vi "do_GB_test.vi"(8 "error in (no error)":errorcluster, 11 "VISA resource name":refnum<visa-resource-name>="COM6") -> (0 "error out":errorcluster, 1 "Results GB":string, 2 "Status GB":string, 3 "VISA resource out":refnum<visa-resource-name>)   [LabVIEW 2015]
doc: "Mini test app for SERIAL RS232 or GPIB communication ports"
uses:
  Type Definitions/Highway_GB_Data.ctl
panel:
  # "Do GB test"
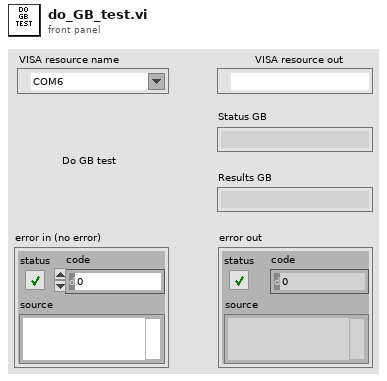
[diagram p1: front panel]
types:
  T1 = typedef "Highway_GB_Data.ctl" = cluster{"Status GB":string, "Results GB":string}
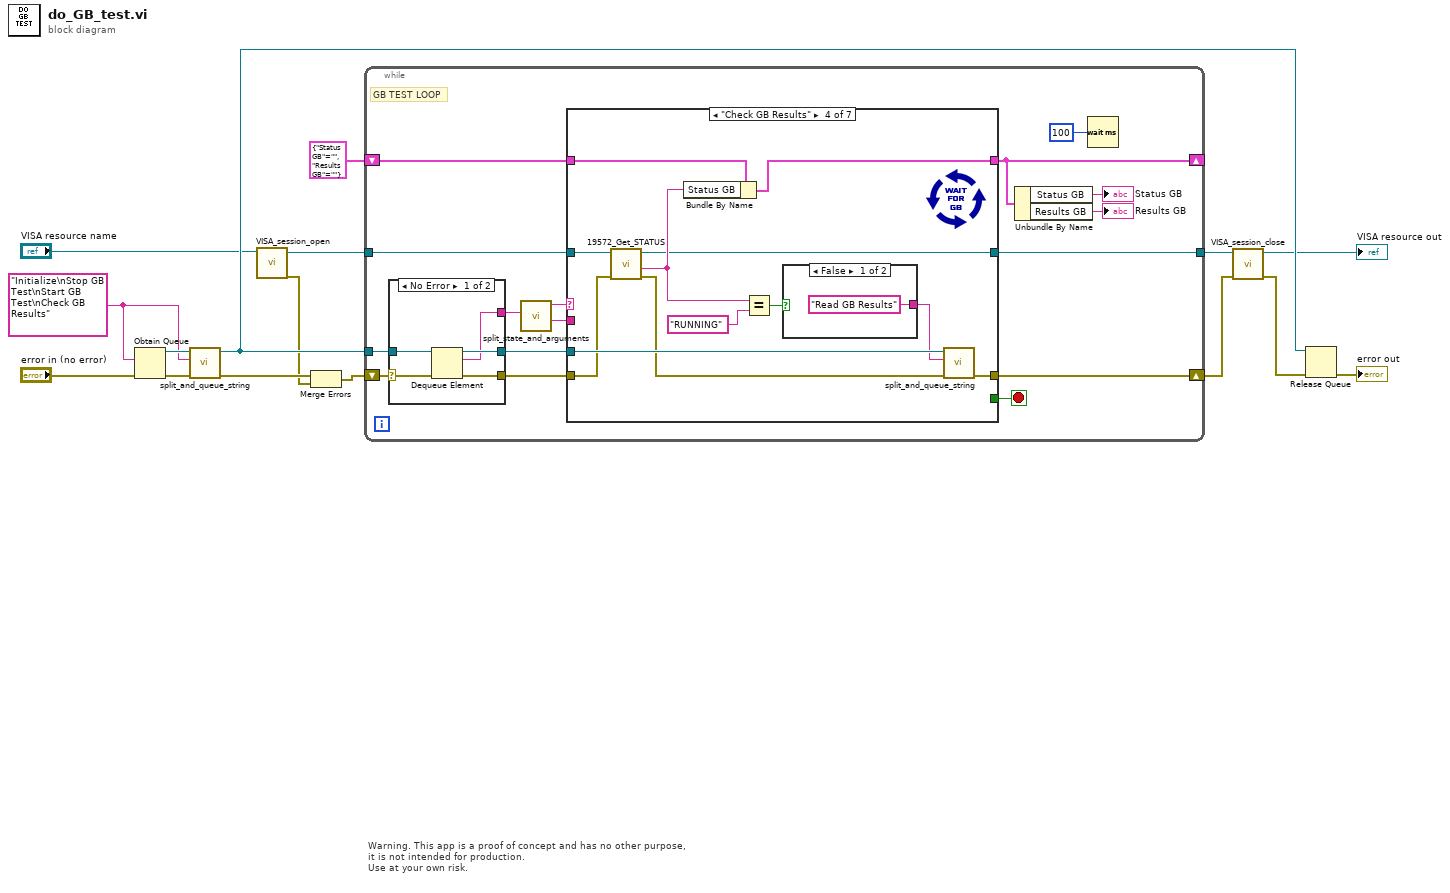
[diagram p0: block diagram]
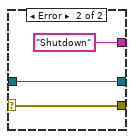
[diagram p2: hidden frame]
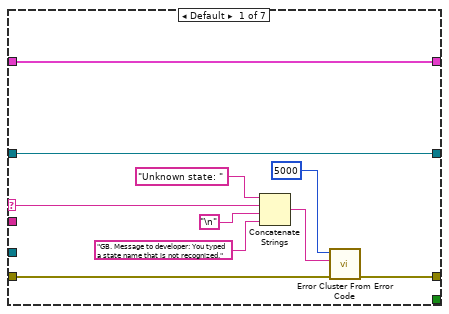
[diagram p3: hidden frame]
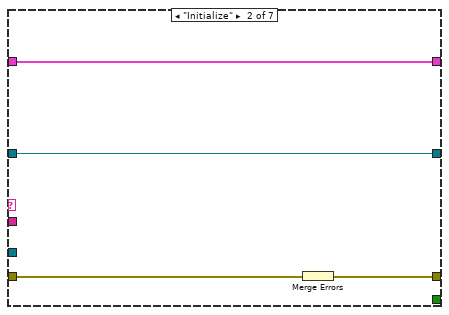
[diagram p4: hidden frame]
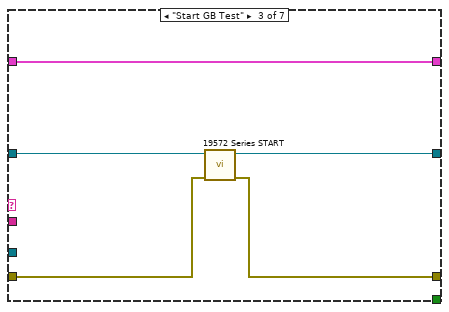
[diagram p5: hidden frame]
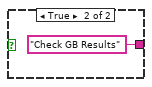
[diagram p6: hidden frame]
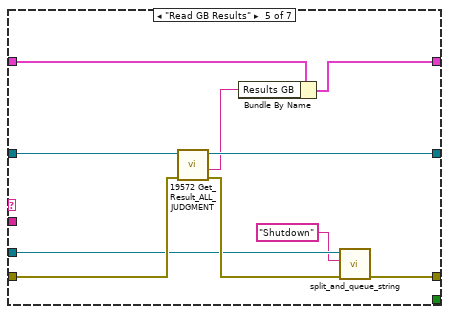
[diagram p7: hidden frame]
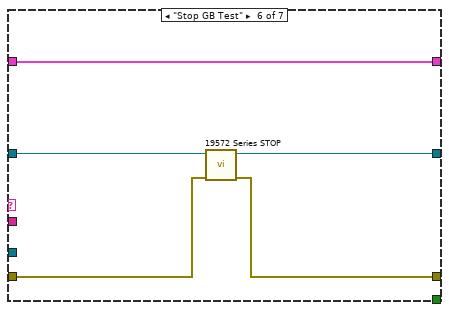
[diagram p8: hidden frame]
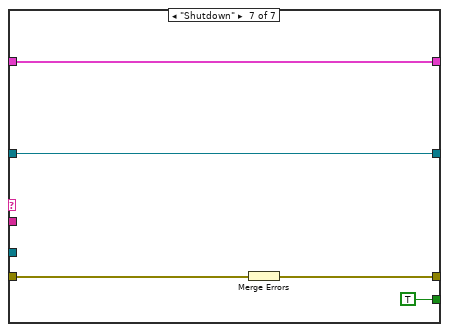
[diagram p9: hidden frame]
diagram:
  w14 = "Initialize\nStop GB Test\nStart GB Test\nCheck GB Results" ("program string")
  # "Warning. This app is a proof of concept and has no other purpose, \nit is not intended for production. \nUse at your own risk."
  n1 = Obtain Queue(element data type=w14, error in (no error)="error in (no error)") -> (queue out=w16:refnum<queue>, error out=w15:errorcluster)  [unwired: 3 in, 1 out]
  n2 = call "split_and_queue_string.vi"("error in (no error)"=w15, "program string"=w14, "queue in"=w16) -> ("error out"=w13:errorcluster, "queue out"=w10:refnum<queue>)  [unwired: 7 in]
  n3 = call "VISA_session_open.vi"("VISA resource name"="VISA resource name") -> ("error out"=w8:errorcluster, "VISA resource name out"=w9:refnum<visa-resource-name>)  [unwired: 9 in]
  n4 = Merge Errors(w13, w8) -> (w11:errorcluster)
  n5 = while {
    shift-right: [w30] -> w6
    shift-left: w11 -> [w23]
    tunnel: w10 -> [w24]
    tunnel: w9 -> [w21]
    shift-right: [w17] -> _
    shift-left: T1 {"Status GB"="", "Results GB"=""} -> [w22]
    tunnel: [w20] -> w7
    stop <- w26 stop-if-true
    # "GB TEST LOOP"
    n6 = case shown="No Error" w23 {
      selector: w23 -> [w37 w40]
      tunnel: [w36 w40] -> w31
      tunnel: w24 -> [w33 w39]
      tunnel: [w35 w39] -> w25
      tunnel: [w34 "Shutdown"] -> w28
      frame No Error {
        n7 = Dequeue Element(queue=w33, error in (no error)=w37) -> (queue out=w35:refnum<queue>, element=w34:string, error out=w36:errorcluster)  [unwired: 1 in, 1 out]
      }
      frame Error {
      }
    }
    n8 = call "split_state_and_arguments.vi"("String"=w28) -> ("Arguments"=w27:string, "State"=w29:string)  [unwired: 9 in]
    n9 = case shown="\"Check GB Results\"" w29 {
      selector: w29 -> [w46 _ _ _ _ _ _]
      tunnel: [w44 w53 w59 w67 w78 w87 w93] -> w30
      tunnel: w31 -> [w45 w52 w58 w70 w83 w88 w92]
      tunnel: w25 -> [_ _ _ w71 w77 _ _]
      tunnel: w27 -> [_ _ _ _ _ _ _]
      tunnel: [_ _ _ _ _ _ TRUE] -> w26
      tunnel: w21 -> [w41 w51 w57 w64 w82 w86 w90]
      tunnel: w22 -> [w42 w54 w56 w63 w81 w85 w89]
      tunnel: [w42 w54 w56 w62 w80 w85 w89] -> w17
      tunnel: [w41 w51 w55 w60 w75 w84 w90] -> w20
      frame Default {
        n10 = Concatenate Strings("Unknown state: " ("string"), w46, "\n", "GB. Message to developer: You typed a state name that is not recognized.") -> (w48:string)
        n11 = call <vilib>:"Error Cluster From Error Code.vi"("error in (no error)"=w45, "error message (\"\")"=w48, "error code (0)"=5000) -> ("error out"=w44:errorcluster)  [unwired: 6 in]
      }
      frame "Initialize" {
        n12 = Merge Errors(w52) -> (w53:errorcluster)
      }
      frame "Start GB Test" {
        n13 = call "19572 Series START.vi"("error in (no error)"=w58, "VISA resource in"=w57) -> ("error out"=w59:errorcluster, "VISA resource out"=w55:refnum<visa-resource-name>)  [unwired: 8 in]
      }
      frame "Check GB Results" {
        n14 = call "19572_Get_STATUS.vi"("error in (no error)"=w70, "VISA resource in"=w64) -> ("error out"=w68:errorcluster, "Status"=w61:string, "VISA resource out"=w60:refnum<visa-resource-name>)  [unwired: 7 in]
        n15 = Bundle By Name(cluster=w63, "Status GB"=w61) -> (w62:T1)
        n16 = Equal?(x=w61, y="RUNNING") -> (x = y?=w65:bool)
        n17 = case shown="False" w65 {
          tunnel: ["Read GB Results" ("program string") "Check GB Results" ("program string")] -> w66
          frame False {
          }
          frame True {
          }
        }
        n18 = call "split_and_queue_string.vi"("error in (no error)"=w68, "program string"=w66, "queue in"=w71) -> ("error out"=w67:errorcluster)  [unwired: 7 in, 1 out]
      }
      frame "Read GB Results" {
        n19 = call "19572 Get_Result_ALL_JUDGMENT.vi"("error in (no error)"=w83, "VISA resource in"=w82) -> ("error out"=w79:errorcluster, "JUDGMENT"=w74:string, "VISA resource out"=w75:refnum<visa-resource-name>)  [unwired: 7 in]
        n20 = Bundle By Name(cluster=w81, "Results GB"=w74) -> (w80:T1)
        n21 = call "split_and_queue_string.vi"("error in (no error)"=w79, "program string"="Shutdown", "queue in"=w77) -> ("error out"=w78:errorcluster)  [unwired: 7 in, 1 out]
      }
      frame "Stop GB Test" {
        n22 = call "19572 Series STOP.vi"("error in (no error)"=w88, "VISA resource in"=w86) -> ("error out"=w87:errorcluster, "VISA resource out"=w84:refnum<visa-resource-name>)  [unwired: 8 in]
      }
      frame "Shutdown" {
        n23 = Merge Errors(w92) -> (w93:errorcluster)
      }
    }
    n24 = Unbundle By Name(w17) -> ("Status GB"=→"Status GB":string, "Results GB"=→"Results GB":string)
    n25 = Wait (ms)(milliseconds to wait=u32 100) -> ()  [unwired: 1 out]
  }
  n26 = call "VISA_session_close.vi"("error in (no error)"=w6, "VISA resource name"=w7) -> ("error out"=w5:errorcluster, "VISA resource out"=→"VISA resource out":refnum<visa-resource-name>)  [unwired: 8 in]
  n27 = Release Queue(queue=w10, error in (no error)=w5) -> (error out=→"error out":errorcluster)  [unwired: 1 in, 2 out]
